vi "数字量输入统计结果.vi"   [LabVIEW 2010]
uses:
  全局量/自动测试结果.vi
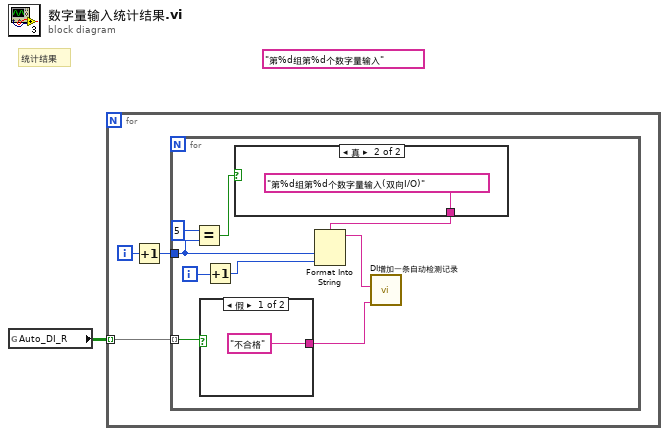
[diagram p0: block diagram]
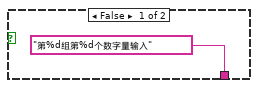
[diagram p2: hidden frame]
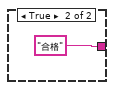
[diagram p3: hidden frame]
diagram:
  (unwired) "第%d组第%d个数字量输入"
  # "统计结果"
  n1 = global read "自动测试结果.vi" "Auto_DI_R"() -> (w1:bool[][])
  n2 = for {
    tunnel: w1 -> [w4] mode=indexing
    i -> [w3]
    n3 = Increment(x=w3) -> (x+1=w2:i32)
    n4 = for {
      tunnel: w4 -> [w10] mode=indexing
      tunnel: w2 -> [w8]
      i -> [w12]
      n5 = Equal?(x=5, y=w8) -> (x = y?=w6:bool)
      n6 = case shown="假" w10 {
        tunnel: ["不合格" "合格"] -> w9
        frame False {
        }
        frame True {
        }
      }
      n7 = Increment(x=w12) -> (x+1=w13:i32)
      n8 = case shown="真" w6 {
        tunnel: ["第%d组第%d个数字量输入" "第%d组第%d个数字量输入(双向I/O)"] -> w5
        frame False {
        }
        frame True {
        }
      }
      n9 = Format Into String(format string=w5, w8, w13) -> (resulting string=w11:string)  [unwired: 2 in, 1 out]
      n10 = call "DI增加一条自动检测记录.vi"("测试结果"=w9, "测试内容"=w11) -> ()  [unwired: 10 in]
    }
  }
